vi "Actor Core.vi"(8 "error in":errorcluster, 11 "Chat Room Controller in":refnum<class "Chat Room Controller.lvclass">) -> (0 "error out":errorcluster, 3 "Actor out":refnum<class "Actor.lvclass">)   [LabVIEW 2025, in "Chat Room Controller.lvlib" / "Chat Room Controller.lvclass"]
doc: "<p>(<strong>Filename</strong>: <span class=\"dnl\">Actor Framework.lvlib:Actor.lvclass:Actor Core.vi</span>)</p>\n<p>Receives messages to the actor, reacts to them, and initiates any error handling that may shut the actor down.</p>\n<p>Descendant classes may override this VI to append parallel tasks for the actor to complete while it handles messages. Overrides use the <a href=\"nihelplauncher://docs/csh?context=lvcore_glang_udclass\">Call Parent Class Method</a> node.</p>"
uses:
  Chat Room Controller.lvclass
  Chat Room Controller.lvclass/Chat Room Controller.ctl
  <vilib>/ActorFramework/Actor/Actor.lvclass
panel:
  out "Message":string
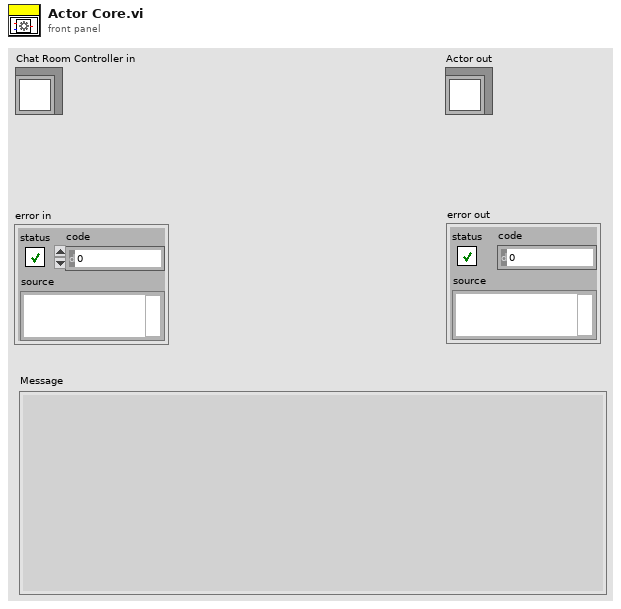
[diagram p1: front panel]
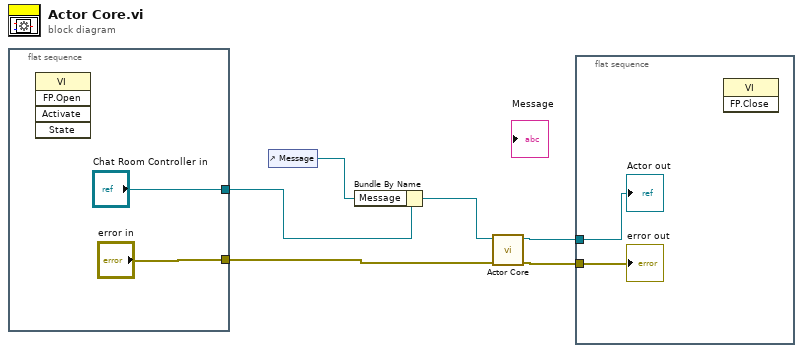
[diagram p0: block diagram]
diagram:
  n1 = flat-sequence {
    tunnel: ["error in"] -> w4
    tunnel: ["Chat Room Controller in"] -> w3
    frame #0 {
      n2 = invoke class="VI" method="FP.Open"() -> ()  [unwired: 5 in, 5 out]
    }
  }
  n3 = control-ref of="Message"() -> (w1:refnum<vi>)
  n4 = Bundle By Name(cluster=w3, "Message"=w1) -> (w2:refnum<class "Chat Room Controller.lvclass">)
  n5 = call-parent "Actor Core.vi"("error in"=w4, "Actor in"=w2) -> ("error out"=w6:errorcluster, "Actor out"=w5:refnum<class "Actor.lvclass">)  [unwired: 8 in]
  n6 = flat-sequence {
    tunnel: w6 -> [w10]
    tunnel: w5 -> [w9]
    frame #0 {
      n7 = invoke class="VI" method="FP.Close"() -> ()  [unwired: 3 in, 3 out]
      "error out" <- w10
      "Actor out" <- w9
    }
  }
